vi "HardwareStart.vi"(8 "Error In":errorcluster, 11 "Keithley 7001 In":refnum<visa-resource-name>) -> (0 "Error Out":errorcluster, 3 "Keithley 7001 Out":refnum<visa-resource-name>)   [LabVIEW 2012]
uses:
  TriggerConfigurationGlobalAction.ctl
  ScanListGlobalAction.ctl
  MemoryGlobalAction.ctl
  driver/Keithley-7001.lvlib
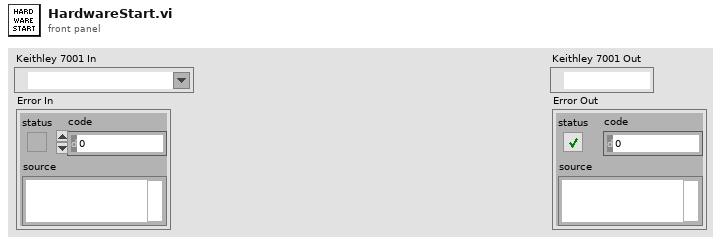
[diagram p1: front panel]
types:
  T1 = typedef "MemoryGlobalAction.ctl" = enum16{"Get", "Set", "Reset"}
  T2 = typedef "ScanListGlobalAction.ctl" = enum16{"Get", "Set", "Reset"}
  T3 = typedef "TriggerConfigurationGlobalAction.ctl" = enum16{"Get", "Set", "Reset"}
  T4 = typedef "TriggerConfiguration.ctl" = cluster{"Arm":T5, "Scan":T7, "Channel":T9}
  T5 = typedef "TriggerArmConfiguration.ctl" = cluster{"Source":T6, "Count":u32, "Infinite?":bool}
  T6 = typedef "Keithley-7001.lvlib/ArmSource.ctl" = enum16{"Hold", "Immediate", "Manual", "Bus", "TLink", "External"}
  T7 = typedef "TriggerScanConfiguration.ctl" = cluster{"Source":T8, "Count":u32, "Infinite?":bool, "Delay (sec)":dbl, "Interval (sec)":dbl}
  T8 = typedef "Keithley-7001.lvlib/ScanSource.ctl" = enum16{"Hold", "Immediate", "Timer", "Manual", "Bus", "TLink", "External"}
  T9 = typedef "TriggerChannelConfiguration.ctl" = cluster{"Source":T10, "Count":u32, "Infinite?":bool, "Auto Count?":bool, "Delay (sec)":dbl, "Interval (sec)":dbl}
  T10 = typedef "Keithley-7001.lvlib/TriggerSource.ctl" = enum16{"Hold", "Immediate", "Manual", "Bus", "TLink", "External", "Timer"}
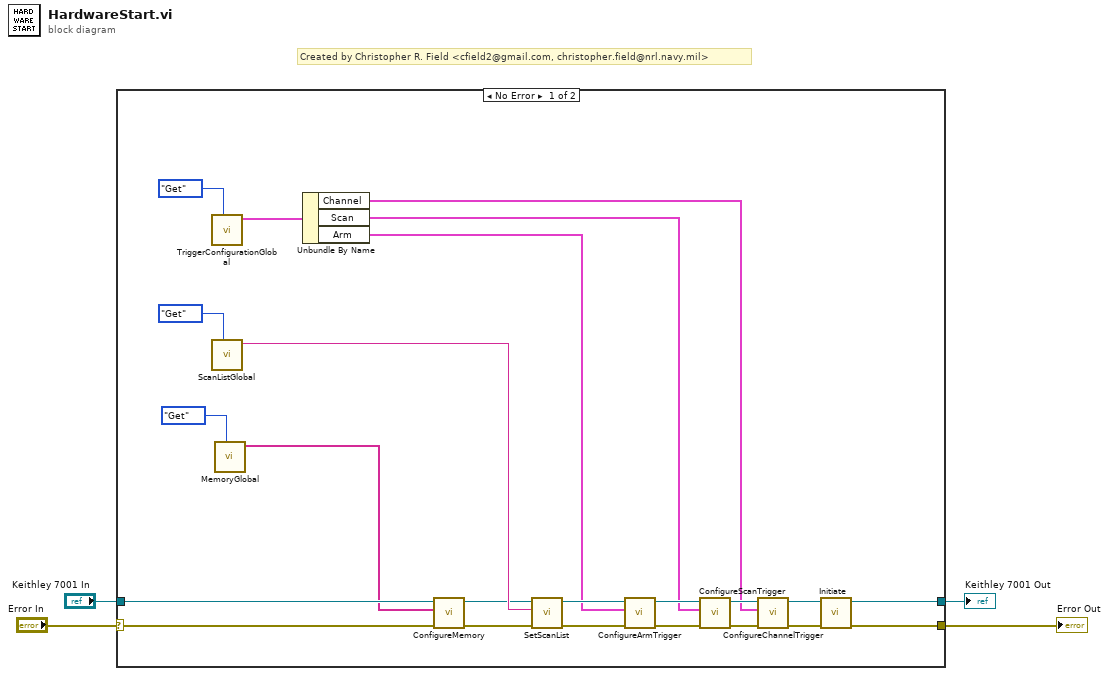
[diagram p0: block diagram]
diagram:
  # "Created by Christopher R. Field <cfield2@gmail.com, christopher.field@nrl.navy.mil>"
  n1 = case shown="No Error" "Error In" {
    selector: "Error In" -> [w6 w28]
    tunnel: "Keithley 7001 In" -> [w7 w29]
    tunnel: [w27 w28] -> w1
    tunnel: [w26 w29] -> w2
    frame No Error {
      n2 = call "TriggerConfigurationGlobal.vi"("Action"=TriggerConfigurationGlobalAction."Get") -> ("Value Out"=w24:T4)  [unwired: 10 in]
      n3 = call "ScanListGlobal.vi"("Action"=ScanListGlobalAction."Get") -> ("Value Out"=w11:string)  [unwired: 10 in]
      n4 = call "MemoryGlobal.vi"("Action"=MemoryGlobalAction."Get") -> ("Value Out"=w5:string[])  [unwired: 10 in]
      n5 = Unbundle By Name(w24) -> ("Channel"=w13:T9, "Scan"=w18:T7, "Arm"=w21:T5)
      n6 = call "ConfigureMemory.vi"("Error In"=w6, "Channel Patterns"=w5, "Keithley 7001 In"=w7) -> ("Error Out"=w8:errorcluster, "Keithley 7001 Out"=w9:refnum<visa-resource-name>)  [unwired: 7 in]
      n7 = call "SetScanList.vi"("Error In"=w8, "Scan List"=w11, "Keithley 7001 In"=w9) -> ("Error Out"=w22:errorcluster, "Keithley 7001 Out"=w23:refnum<visa-resource-name>)  [unwired: 7 in]
      n8 = call "ConfigureArmTrigger.vi"("Error In"=w22, "Arm Configuration"=w21, "Keithley 7001 In"=w23) -> ("Error Out"=w19:errorcluster, "Keithley 7001 Out"=w20:refnum<visa-resource-name>)  [unwired: 7 in]
      n9 = call "ConfigureScanTrigger.vi"("Error In"=w19, "Scan Configuration"=w18, "Keithley 7001 In"=w20) -> ("Error Out"=w16:errorcluster, "Keithley 7001 Out"=w17:refnum<visa-resource-name>)  [unwired: 7 in]
      n10 = call "ConfigureChannelTrigger.vi"("Error In"=w16, "Channel Configuration"=w13, "Keithley 7001 In"=w17) -> ("Error Out"=w14:errorcluster, "Keithley 7001 Out"=w15:refnum<visa-resource-name>)  [unwired: 7 in]
      n11 = call "Initiate.vi"("Error In"=w14, "Keithley 7001 In"=w15) -> ("Error Out"=w27:errorcluster, "Keithley 7001 Out"=w26:refnum<visa-resource-name>)  [unwired: 8 in]
    }
    frame Error {
    }
  }
  "Keithley 7001 Out" <- w2
  "Error Out" <- w1
